vi "cblas drotm.vi"(5 "n":i32=-1, 6 "incy":i32=1, 7 "incx":i32=1, 8 "Rotation Matrix":T1, 9 "flag":i32(ring)=-1 items=["-2"=-2, "-1"=-1, "0"=0, "1"=1], 10 "y in":dbl[](array[numeric]), 11 "x in":dbl[](array[numeric])) -> (0 "error":i32, 2 "y out":dbl[](array[numeric]), 3 "x out":dbl[](array[numeric]))   [LabVIEW 2017, in "NI_AALBLAS.lvlib"]
uses:
  <vilib>/Analysis/NI_AALBLAS.lvlib
  <vilib>/Analysis/Matrix/Datatypes/RealMatrix.ctl
  <resource>/lvblas.dll
  <vilib>/Analysis/Matrix/NI_Matrix.lvlib
panel:
  # "void cblas_drotm(n, *x, incx, *y, incy, *Rotation)"
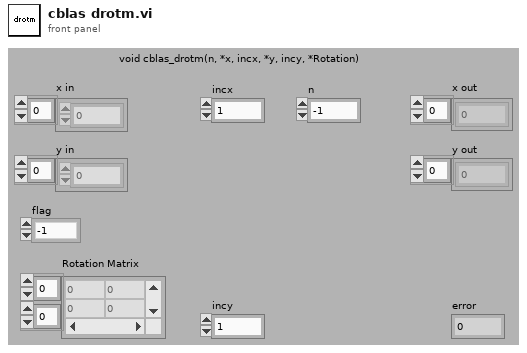
[diagram p1: front panel]
types:
  T1 = typedef "NI_Matrix.lvlib/RealMatrix.ctl" = dbl[][]
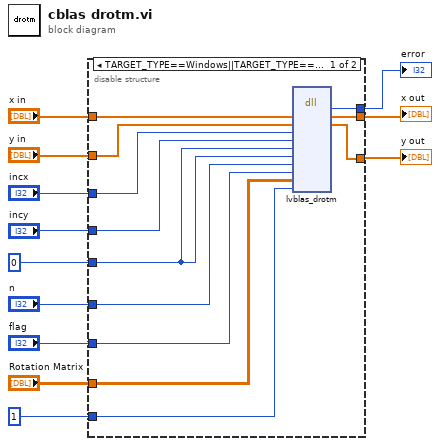
[diagram p0: block diagram]
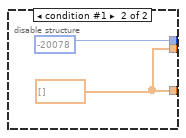
[diagram p2: hidden frame]
diagram:
  n1 = disable-structure shown="TARGET_TYPE==Windows||TARGET_TYPE==Unix||TARGET_TYPE==RT||TARGET_TYPE==Mac" {
    disable-tunnel: "x in" -> [w24 _]
    disable-tunnel: "y in" -> [w23 _]
    disable-tunnel: "n" -> [w22 _]
    disable-tunnel: [w21 -20078] -> w9
    disable-tunnel: 0 -> [w20 _]
    disable-tunnel: [w19 w25] -> w7
    disable-tunnel: [w18 w25] -> w6
    disable-tunnel: "incx" -> [w17 _]
    disable-tunnel: "incy" -> [w16 _]
    disable-tunnel: "flag" -> [w15 _]
    disable-tunnel: "Rotation Matrix" -> [w14 _]
    disable-tunnel: 1 -> [w13 _]
    frame condition #0 (active) {
      n2 = dll-call lib="e:/builds/penguin/labview/branches/2017/dev/dist/resource/lvblas.*" fn="lvblas_drotm" ("CBLAS.dll:DotProdH")("X"=w24, "Y"=w23, "IncX"=w17, "IncY"=w16, "startX"=w20, "startY"=w20, "N"=w22, "flag"=w15, "Rotation"=w14, "check"=w13) -> ("error"=w21:i32, "X"=w19:dbl[], "Y"=w18:dbl[])  [unwired: 11 in, 2 out]
    }
    frame condition #1 {
      w25 = dbl[] []
    }
  }
  "error" <- w9
  "x out" <- w7
  "y out" <- w6
